vi "MEMR-Compute Gain.vi"(0 "Test":dbl[](array[numeric]), 2 "PT":cluster{"Freq":dbl[], "Mag":dbl[]}, 5 "Baseline":dbl[](array[numeric]), 7 "Fs (Hz)":dbl format="%#_13g", 9 "Analysis":T2) -> (4 "spectra":cluster{"Freq (Hz)":dbl[], dbl[][]}, 6 "gain spectrum":T1, 8 "Gain (dB)":dbl)   [LabVIEW 2020]
uses:
  Typedefs/MEMR-Analysis.ctl
  <vilib>/Analysis/4window.llb/Hanning Window (DBL).vi
  <vilib>/Analysis/4window.llb/Hamming Window (DBL).vi
  <vilib>/Analysis/baseanly.llb/Mean (DBL).vi
  <vilib>/Analysis/4window.llb/AllCosWindow (DBL).vi
  Utility VIs/Math VIs/FFT x(t) to dB,Degrees (1D).vi
  Utility VIs/Math VIs/interp1 (1D).vi
  Utility VIs/Array Manipulation VIs/Irregular Array Subset (DBL).vi
  Utility VIs/Math VIs/dB to Linear (1D).vi
  Utility VIs/Math VIs/Linear to dB (scalar).vi
  <vilib>/Analysis/NI_AALPro.lvlib
  <vilib>/Analysis/NI_AALBase.lvlib
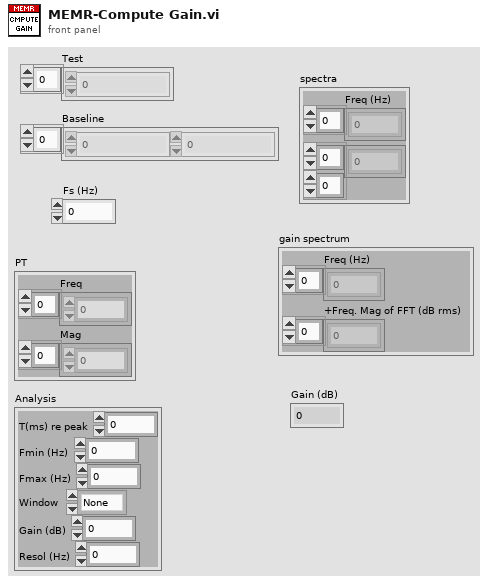
[diagram p1: front panel]
types:
  T1 = cluster{"Freq (Hz)":dbl[], "+Freq. Mag of FFT (dB rms)":dbl[]}
  T2 = typedef "MEMR-Analysis.ctl" = cluster{"T(ms) re peak":dbl, "Fmin (Hz)":dbl, "Fmax (Hz)":dbl, "Window":enum16{"None", "Hanning", "Hamming"}, "Gain (dB)":dbl, "Resol (Hz)":dbl}
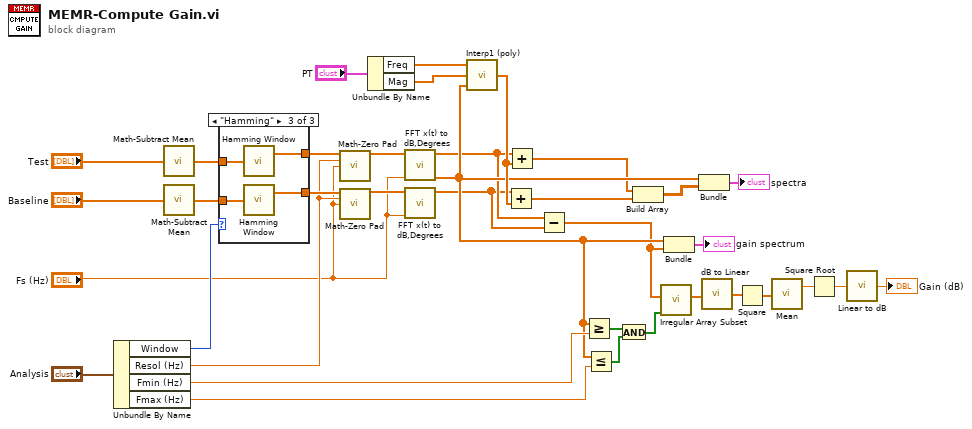
[diagram p0: block diagram]
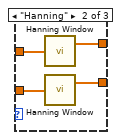
[diagram p3: hidden frame]
diagram:
  n1 = Unbundle By Name("Analysis") -> ("Window"=w34:enum16{"None", "Hanning", "Hamming"}, "Resol (Hz)"=w10:dbl, "Fmin (Hz)"=w33:dbl, "Fmax (Hz)"=w32:dbl)
  n2 = call "Math-Subtract Mean.vi"("Y"="Test") -> ("Y - mean(Y)"=w16:dbl[])  [unwired: 4 in]
  n3 = call "Math-Subtract Mean.vi"("Y"="Baseline") -> ("Y - mean(Y)"=w15:dbl[])  [unwired: 4 in]
  n4 = case shown="\"Hamming\"" w34 {
    tunnel: w16 -> [w38 w42 w46]
    tunnel: w15 -> [w37 w39 w44]
    tunnel: [w38 w41 w45] -> w12
    tunnel: [w37 w40 w43] -> w14
    frame "None", Default {
    }
    frame "Hanning" {
      n5 = call-poly <vilib>:"Hanning Window.vi"("X"=w42) -> ("Windowed X"=w41:dbl[])  [unwired: 1 out]
      n6 = call-poly <vilib>:"Hanning Window.vi"("X"=w39) -> ("Windowed X"=w40:dbl[])  [unwired: 1 out]
    }
    frame "Hamming" {
      n7 = call-poly <vilib>:"Hamming Window.vi"("X"=w46) -> ("Windowed X"=w45:dbl[])  [unwired: 1 out]
      n8 = call-poly <vilib>:"Hamming Window.vi"("X"=w44) -> ("Windowed X"=w43:dbl[])  [unwired: 1 out]
    }
  }
  n9 = call "Math-Zero Pad.vi"("Signal"=w12, "Resol (Hz)"=w10, "Fs (Hz)"="Fs (Hz)") -> ("Zero-padded signal"=w11:dbl[])  [unwired: 11 in, 1 out]
  n10 = call "Math-Zero Pad.vi"("Signal"=w14, "Resol (Hz)"=w10, "Fs (Hz)"="Fs (Hz)") -> ("Zero-padded signal"=w13:dbl[])  [unwired: 11 in, 1 out]
  n11 = Unbundle By Name("PT") -> ("Freq"=w23:dbl[], "Mag"=w22:dbl[])
  n12 = call-poly "FFT x(t) to dB,Degrees.vi"("Fs (Hz)"="Fs (Hz)", "X"=w11) -> ("Freq (Hz)"=w19:dbl[], "+Freq. Mag of FFT (dB rms)"=w3:dbl[])  [unwired: 7 in, 1 out]
  n13 = call-poly "FFT x(t) to dB,Degrees.vi"("Fs (Hz)"="Fs (Hz)", "X"=w13) -> ("+Freq. Mag of FFT (dB rms)"=w2:dbl[])  [unwired: 7 in, 2 out]
  n14 = call-poly "Interp1 (poly).vi"("X"=w23, "Y"=w22, "U"=w19) -> ("V"=w21:dbl[])  [unwired: 2 in]
  n15 = Add(x=w2, y=w21) -> (x+y=w17:dbl[])
  n16 = Add(x=w3, y=w21) -> (x+y=w18:dbl[])
  n17 = Subtract(x=w3, y=w2) -> (x-y=w1:dbl[])
  n18 = Greater Or Equal?(x=w19, y=w33) -> (x >= y?=w31:bool[])
  n19 = Less Or Equal?(x=w19, y=w32) -> (x <= y?=w30:bool[])
  n20 = And(x=w31, y=w30) -> (x .and. y?=w29:bool[])
  n21 = Build Array(w18, w17) -> (w20:dbl[][])
  n22 = call-poly "Irregular Array Subset.vi"("Mask"=w29, "Array"=w1) -> ("Array Subset"=w28:dbl[])  [unwired: 8 in, 1 out]
  n23 = Bundle("Freq (Hz)"=w19, w1) -> (→"gain spectrum":cluster{"Freq (Hz)":dbl[], dbl[]})  [unwired: 1 in]
  n24 = Bundle("Freq (Hz)"=w19, w20) -> (→"spectra":cluster{"Freq (Hz)":dbl[], dbl[][]})  [unwired: 1 in]
  n25 = call-poly "dB to Linear.vi"("dB"=w28) -> ("linear"=w27:dbl[])
  n26 = Square(x=w27) -> (x^2=w26:dbl[])
  n27 = call-poly <vilib>:"Mean.vi"("X"=w26) -> ("mean"=w25:dbl)  [unwired: 1 out]
  n28 = Square Root(x=w25) -> (sqrt(x)=w24:dbl)
  n29 = call-poly "Linear to dB.vi"("Linear"=w24) -> ("dB"=→"Gain (dB)":dbl)
